vi "Init.vi"(8 "error in (no error)":errorcluster caption="entrée d'erreur (pas d'erreur)", 11 "Class UART (Default) en entrée":refnum<class "Class UART (Default).lvclass">) -> (0 "error out":errorcluster caption="sortie d'erreur", 3 "Class UART (Default) en sortie":refnum<class "Class UART (Default).lvclass">)   [LabVIEW 2020, in "Library Instrument & Equipement.lvlib" / "Library UART.lvlib" / "Class UART (Default).lvclass"]
uses:
  Class UART (Default).lvclass
  Class UART (Default).lvclass/Class UART (Default).ctl
  <vilib>/Instr/_visa.llb/VISA Configure Serial Port (Instr).vi
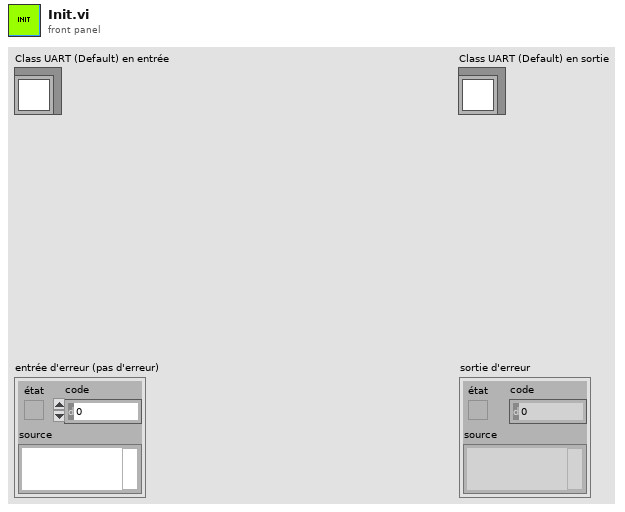
[diagram p1: front panel]
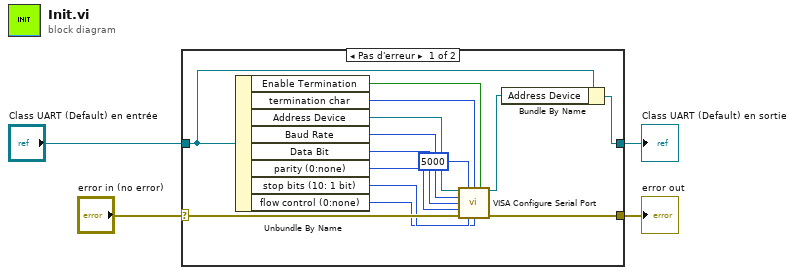
[diagram p0: block diagram]
diagram:
  n1 = case shown="Pas d'erreur" "error in (no error)" {
    selector: "error in (no error)" -> [w18 w20]
    tunnel: [w17 w20] -> w3
    tunnel: [w12 w19] -> w1
    tunnel: "Class UART (Default) en entrée" -> [w13 w19]
    frame No Error {
      n2 = Unbundle By Name(w13) -> ("Enable Termination"=w14:bool, "termination char"=w15:u8, "Address Device"=w16:refnum<visa-resource-name>, "Baud Rate"=w10:u32, "Data Bit"=w9:u16, "parity (0:none)"=w8:enum16{"None", "Odd", "Even", "Mark", "Space"}, "stop bits (10: 1 bit)"=w7:u16, "flow control (0:none)"=w6:u16)
      n3 = call-poly "VISA Configure Serial Port"("VISA resource name"=w16, "timeout (10sec)"=u32 5000, "termination char\n(0xA = '\\n' = LF)"=w15, "Enable Termination\nChar (T)"=w14, "baud rate (9600)"=w10, "data bits (8)"=w9, "parity (0:none)"=w8, "error in (no error)"=w18, "stop bits (10: 1 bit)"=w7, "flow control (0:none)"=w6) -> ("VISA resource name out"=w11:refnum<visa-resource-name>, "error out"=w17:errorcluster)  [unwired: 4 in]
      n4 = Bundle By Name(cluster=w13, "Address Device"=w11) -> (w12:refnum<class "Class UART (Default).lvclass">)
    }
    frame Error {
    }
  }
  "error out" <- w3
  "Class UART (Default) en sortie" <- w1
